vi "CgtpRunProgram.vi"(8 "lineNum":i32, 9 "progName":string, 10 "Cgtp":refnum<k24>, 11 "error in":errorcluster) -> (3 "error out":errorcluster)   [LabVIEW 2016, in "UnderAutomation.Fanuc.lvlib"]
uses:
  UnderAutomation.Fanuc.lvlib
  C:/Users/fg/Documents/Fanuc.vi/LabVIEW_2024/UnderAutomation.Fanuc/lib/UnderAutomation.Fanuc.dll
  LabVIEW_2024/UnderAutomation.Fanuc/lib/UnderAutomation.Fanuc.dll
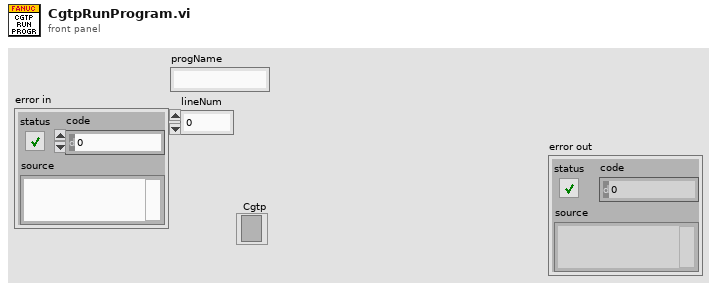
[diagram p1: front panel]
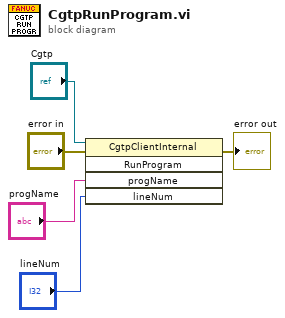
[diagram p0: block diagram]
diagram:
  n1 = invoke class="CgtpClientInternal" method="RunProgram"(reference="Cgtp", error in="error in", "progName"="progName", "lineNum"="lineNum") -> (error out=→"error out":errorcluster)  [unwired: 1 in, 4 out]
